vi "Set Volt Mode.vi"(8 "error in (no error)":errorcluster, 11 "Async Data in":T1={"Hardware"={"Switch Device"="", "DMM Device"="", "DMM -> Switch Trigger"=0, "Switch -> DMM Trigger"=0, "Sample Interval (sec)"=0.0, "Current Samples"=0, "Current Limit"=1.2, "Current Resolution"=5.5, "Auto-Read"=FALSE, "Keep Values"=FALSE}, "Communication"={"Status Q"=refnum, "Command Q"=refnum, "Voltage FIFO"=refnum, "Voltage Buffer"=[], "Current FIFO"=refnum, "Current Buffer"=[], "Async Events"=refnum}} {"Hardware"."Current Resolution" items=["3 1/2"=3.5, "4 1/2"=4.5, "5 1/2"=5.5, "6 1/2"=6.5, "7 1/2"=7.5]; "Hardware"."Sample Interval (sec)" format="%.2f"}) -> (0 "error out":errorcluster)   [LabVIEW 2011, in "Switch-DMM Custom Device.lvlib"]
uses:
  Switch-DMM Custom Device.lvlib
  Controls/Async Data.ctl
  Controls/Hardware.ctl
  <instrlib>/niDMM/nidmm.llb/niDMM Resolution in Digits.ctl
  Controls/Communication.ctl
  Controls/Async Status.ctl
  Controls/Async State.ctl
  Controls/Async Command.ctl
  Controls/Async Events.ctl
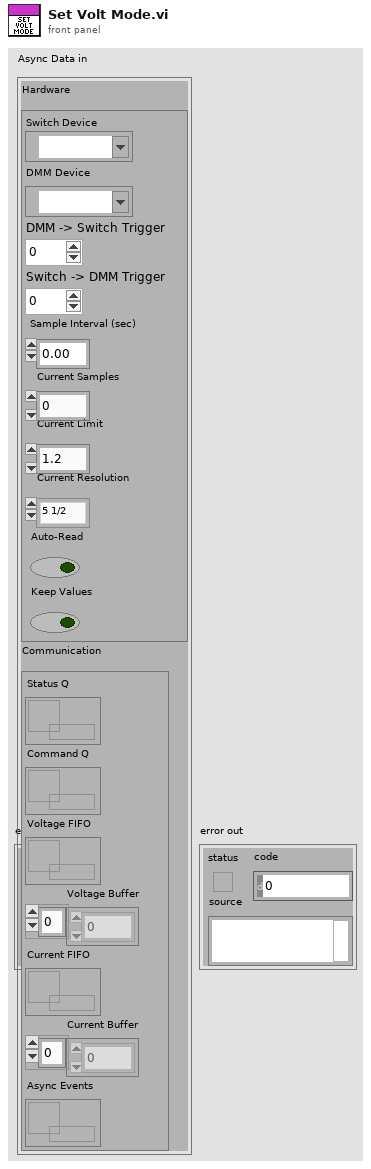
[diagram p1: front panel]
types:
  T1 = typedef "Switch-DMM Custom Device.lvlib/Async Data.ctl" = cluster{"Hardware":T2, "Communication":T4}
  T2 = typedef "Switch-DMM Custom Device.lvlib/Hardware.ctl" = cluster{"Switch Device":refnum<k15>, "DMM Device":refnum<k15>, "DMM -> Switch Trigger":u16, "Switch -> DMM Trigger":u16, "Sample Interval (sec)":dbl, "Current Samples":i32, "Current Limit":dbl, "Current Resolution":T3, "Auto-Read":bool, "Keep Values":bool}
  T3 = typedef "niDMM Resolution in Digits.ctl" = dbl
  T4 = typedef "Switch-DMM Custom Device.lvlib/Communication.ctl" = cluster{"Status Q":refnum<queue>, "Command Q":refnum<queue>, "Voltage FIFO":refnum<k33>, "Voltage Buffer":dbl[], "Current FIFO":refnum<k33>, "Current Buffer":dbl[], "Async Events":refnum<queue>}
  T5 = typedef "Switch-DMM Custom Device.lvlib/Async Command.ctl" = enum16{"None", "Start", "Set Cur Mode", "Req Volt Mode", "Set Volt Mode", "Read Volt", "Exit"}
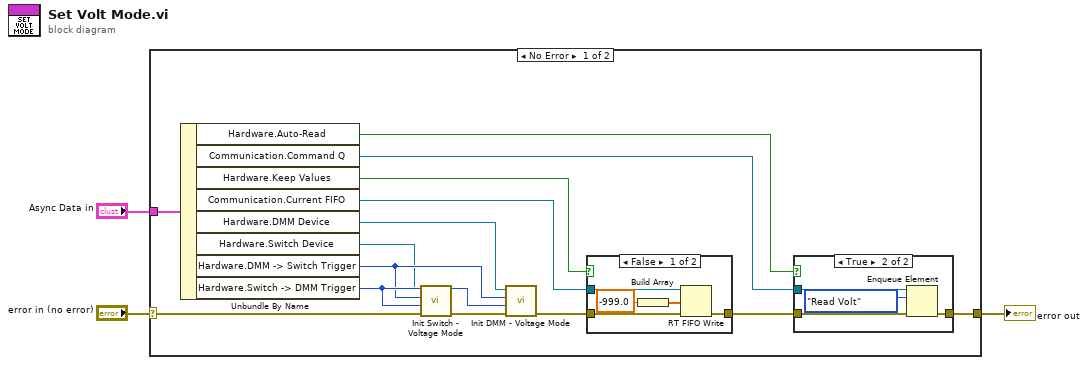
[diagram p0: block diagram]
diagram:
  n1 = case shown="No Error" "error in (no error)" {
    selector: "error in (no error)" -> [w9 w29]
    tunnel: [w16 w29] -> w3
    tunnel: "Async Data in" -> [w10 _]
    frame No Error {
      n2 = Unbundle By Name(w10) -> ("Hardware.Auto-Read"=w8:bool, "Communication.Command Q"=w17:refnum<queue>, "Hardware.Keep Values"=w4:bool, "Communication.Current FIFO"=w6:refnum<k33>, "Hardware.DMM Device"=w12:refnum<k15>, "Hardware.Switch Device"=w11:refnum<k15>, "Hardware.DMM -> Switch Trigger"=w13:u16, "Hardware.Switch -> DMM Trigger"=w14:u16)
      n3 = call "Init Switch - Voltage Mode.vi"("error in (no error)"=w9, "Switch -> DMM Trigger"=w14, "DMM -> Switch Trigger"=w13, "Switch Device in"=w11) -> ("error out"=w15:errorcluster)  [unwired: 6 in, 1 out]
      n4 = call "Init DMM - Voltage Mode.vi"("error in (no error)"=w15, "Switch -> DMM Trigger"=w14, "DMM -> Switch Trigger"=w13, "DMM Device in"=w12) -> ("error out"=w7:errorcluster)  [unwired: 6 in, 1 out]
      n5 = case shown="False" w4 {
        tunnel: w7 -> [w22 w23]
        tunnel: w6 -> [w21 _]
        tunnel: [w18 w23] -> w5
        frame False {
          n6 = Build Array(-999.0) -> (w19:dbl[])
          n7 = RT FIFO Write(0:w21, 1:w19, 3:w22) -> (11:w18:errorcluster)  [unwired: 2 in, 3 out]
        }
        frame True {
        }
      }
      n8 = case shown="True" w8 {
        tunnel: w17 -> [_ w28]
        tunnel: [w24 w27] -> w16
        tunnel: w5 -> [w24 w25]
        frame False {
        }
        frame True {
          n9 = Enqueue Element(queue=w28, element=Async_Command."Read Volt", error in (no error)=w25) -> (error out=w27:errorcluster)  [unwired: 1 in, 2 out]
        }
      }
    }
    frame Error {
    }
  }
  "error out" <- w3
